vi "retrieveConfiguration.vi"(8 "error in (no error)":errorcluster, 10 "configName":string) -> (0 "error out":errorcluster, 2 "xmlData":string)   [LabVIEW 2013]
uses:
  <userlib>/Common/ConfigurationReader/ConfigurationReader.lvclass
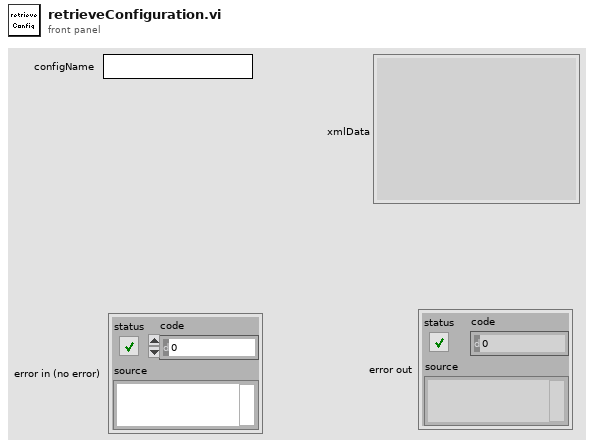
[diagram p1: front panel]
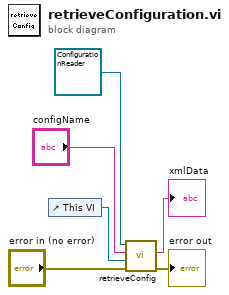
[diagram p0: block diagram]
diagram:
  n1 = control-ref of="This VI"() -> (w4:refnum<vi>)
  n2 = call <userlib>:"retrieveConfig.vi"("error in (no error)"="error in (no error)", "callingVIRef"=w4, "configName"="configName", "ConfigurationReader in"=refnum<class "ConfigurationReader.lvclass"> refnum) -> ("error out"=→"error out":errorcluster, "xmlData"=→"xmlData":string)  [unwired: 5 in, 1 out]
